vi "FINDING A RANDOM NUMBER.vi"() -> ()   [LabVIEW 2018]
panel:
  out "size(s)":i32
  in  "USER INPUT":dbl
  # "FINDING A RANDOM NUMBER"
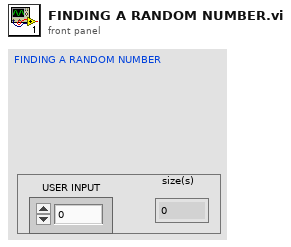
[diagram p1: front panel]
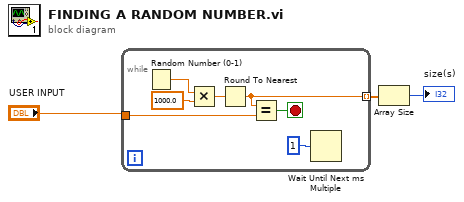
[diagram p0: block diagram]
diagram:
  n1 = while {
    tunnel: "USER INPUT" -> [w6]
    tunnel: [w4] -> w2 mode=indexing
    stop <- w7 stop-if-true
    n2 = Random Number (0-1)() -> (number: 0 to 1=w10:dbl)
    n3 = Multiply(x=w10, y=1000.0) -> (x*y=w8:dbl)
    n4 = Round To Nearest(number=w8) -> (nearest integer value=w4:dbl)
    n5 = Equal?(x=w4, y=w6) -> (x = y?=w7:bool)
    n6 = Wait Until Next ms Multiple(millisecond multiple=u32 1) -> ()  [unwired: 1 out]
  }
  n7 = Array Size(array=w2) -> (size(s)=→"size(s)":i32)
